vi "Sub Initialize.vi"(8 "error in (no error)":errorcluster, 11 "Instrument Recorder in":refnum<class "Line Detector.lvclass">) -> (0 "error out":errorcluster, 2 "Initialize Result":refnum<class "Acquired Result.lvclass">, 3 "Instrument Recorder out":refnum<class "Line Detector.lvclass">)   [LabVIEW 2016, in "Line Detector.lvclass"]
uses:
  Line Detector.lvclass
  C:/Program Files (x86)/National Instruments/LabVIEW 2016/vi.lib/ActorFramework/Actor/Actor.lvclass
  Results/Acquired Result/Acquired Result.lvclass
  Line Detector.lvclass/Line Detector.ctl
  <vilib>/ActorFramework/Actor/Actor.lvclass/Actor.ctl
  <vilib>/ActorFramework/Message Enqueuer/Message Enqueuer.lvclass/Message Enqueuer.ctl
  Template Module Messages/Subscribe Request Msg/Subscribe Request Msg.lvclass/Subscribe Request Msg.ctl
  <vilib>/ActorFramework/Message Enqueuer/Init from Existing Queue.vi
  <vilib>/ActorFramework/Message Enqueuer/Enqueue.vi
  Template Module Messages/Subscribe Request Msg/Subscribe Request Msg.lvclass
  C:/Program Files (x86)/National Instruments/LabVIEW 2016/vi.lib/ActorFramework/Message/Message.lvclass
  Read Line detector configuration.vi
  <vilib>/ActorFramework/Message Priority Queue/Priority Enqueue.vi
  Process Object/Process Object.lvclass
  <vilib>/ActorFramework/Message Enqueuer/Message Enqueuer.lvclass
  <vilib>/ActorFramework/Actor/Actor.lvclass
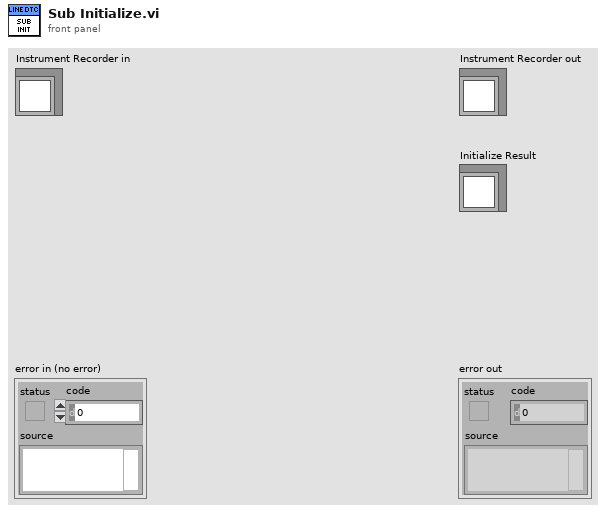
[diagram p1: front panel]
types:
  T1 = typedef "Line Detector Configuration.ctl" = cluster{"Peak width guess":dbl, "Background removal":enum16{"NONE", "High-pass", "Detrend"}, "Smoothing":enum16{"NONE", "Low-pass", "Denoise"}, "Smooth window":dbl, "Relative threshold":dbl, "Peak detector":enum16{"Normal", "Wavelet", "Wavelet+detrend"}, "Bgd window":dbl, "Spectrum recorder name":string, "Fit window":dbl}
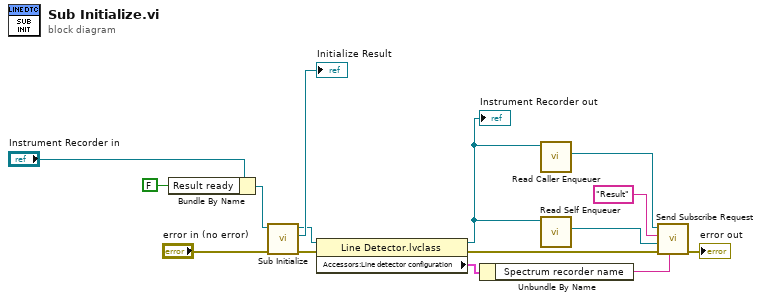
[diagram p0: block diagram]
diagram:
  n1 = Bundle By Name(cluster="Instrument Recorder in", "Result ready"=FALSE) -> (w2:refnum<class "Line Detector.lvclass">)
  n2 = call-parent "Sub Initialize.vi"("error in (no error)"="error in (no error)", "Instrument Recorder in"=w2) -> ("error out"=w11:errorcluster, "Initialize Result"=→"Initialize Result":refnum<class "Acquired Result.lvclass">, "Instrument Recorder out"=w6:refnum<class "Line Detector.lvclass">)  [unwired: 7 in]
  n3 = property class="Line Detector.lvclass"(reference=w6, error in=w11) -> (reference out=w3:refnum<class "Line Detector.lvclass">, error out=w7:errorcluster, "Accessors:Line detector configuration"=w5:T1)
  "Instrument Recorder out" <- w3
  n4 = Unbundle By Name(w5) -> ("Spectrum recorder name"=w4:string)
  n5 = call <vilib>:"Read Caller Enqueuer.vi"("Actor"=w3) -> ("Caller Enqueuer"=w9:refnum<class "Message Enqueuer.lvclass">)  [unwired: 10 in]
  n6 = call <vilib>:"Read Self Enqueuer.vi"("Actor"=w3) -> ("Self Enqueuer"=w8:refnum<class "Message Enqueuer.lvclass">)  [unwired: 10 in]
  n7 = call "Send Subscribe Request.vi"("Broadcaster"=w4, "error in (no error)"=w7, "Subscriber Enqueuer"=w8, "Topic"="Result", "Message Enqueuer"=w9) -> ("error out"=→"error out":errorcluster)  [unwired: 5 in, 1 out]
